vi "calc FFT_indexed.vi"(6 "#bins":i32, 7 "IQ indexes":i32[][](array[numeric]), 8 "dt":dbl=1e-06 format="%#_13g", 9 "Unit":T1, 10 "Window":T2=1 items=["Rectangle"=0, "Hanning"=1, "Hamming"=2, "Blackman-Harris"=3, "Exact Blackman"=4, "Blackman"=5, "Flat Top"=6, "4 Term B-Harris "=7, "7 Term B-Harris"=8, "Low Sidelobe"=9, "Blackman Nuttall"=11, "Triangle"=30, "Bartlett-Hanning"=31, "Bohman"=32, "Parzen"=33, "Welch"=34, "Kaiser"=60, "Dolph-Chebyshev"=61, "Gaussian"=62], 11 "data":dbl[][](array[numeric])) -> (3 "Power Spectrum / PSD":cluster{"f0":dbl, "df":dbl, "magnitude":dbl[]}[](array[cluster]) {"magnitude" format="%.2p"; "f0" format="%.2p"; "df" format="%.2p"})   [LabVIEW 2018]
uses:
  <vilib>/Analysis/4window.llb/windowTd.ctl
  controls/power_spectrum_unit.ctl
  <vilib>/measure/maspectr.llb/Power Spectrum and PSD Export Mode.ctl
  <vilib>/Analysis/0measdsp.llb/Scaled Time Domain Window (DBL).vi
  <vilib>/measure/maspectr.llb/FFT Power Spectrum and PSD for N Chan (CDB).vi
  <vilib>/measure/NI_MAPro.lvlib
  <vilib>/Analysis/NI_AALPro.lvlib
panel:
  # "each row is a pair of indexes in the data matrix.\nThe first index is I of that channelm the second is Q of that channel"
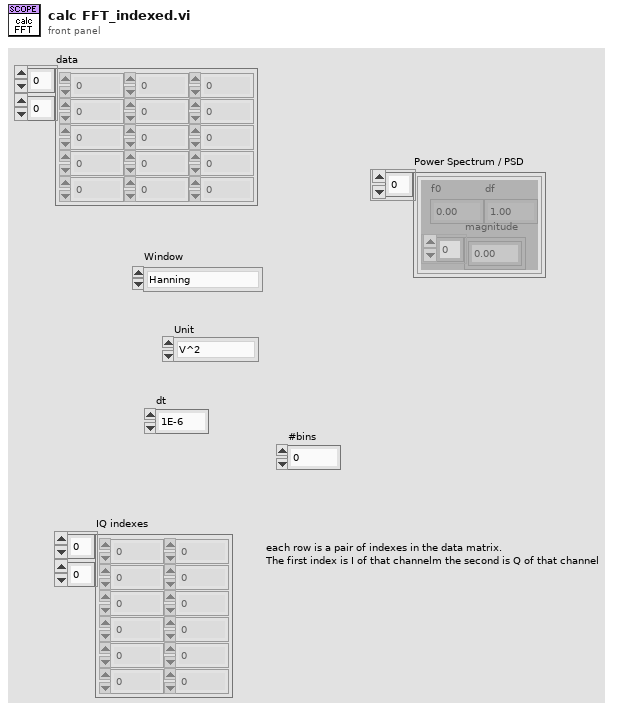
[diagram p1: front panel]
types:
  T1 = typedef "power_spectrum_unit.ctl" = enum16{"V^2", "V", "dBV"}
  T2 = typedef "NI_AALPro.lvlib/windowTd.ctl" = u32
  T3 = typedef "NI_MAPro.lvlib/Power Spectrum and PSD Export Mode.ctl" = u16
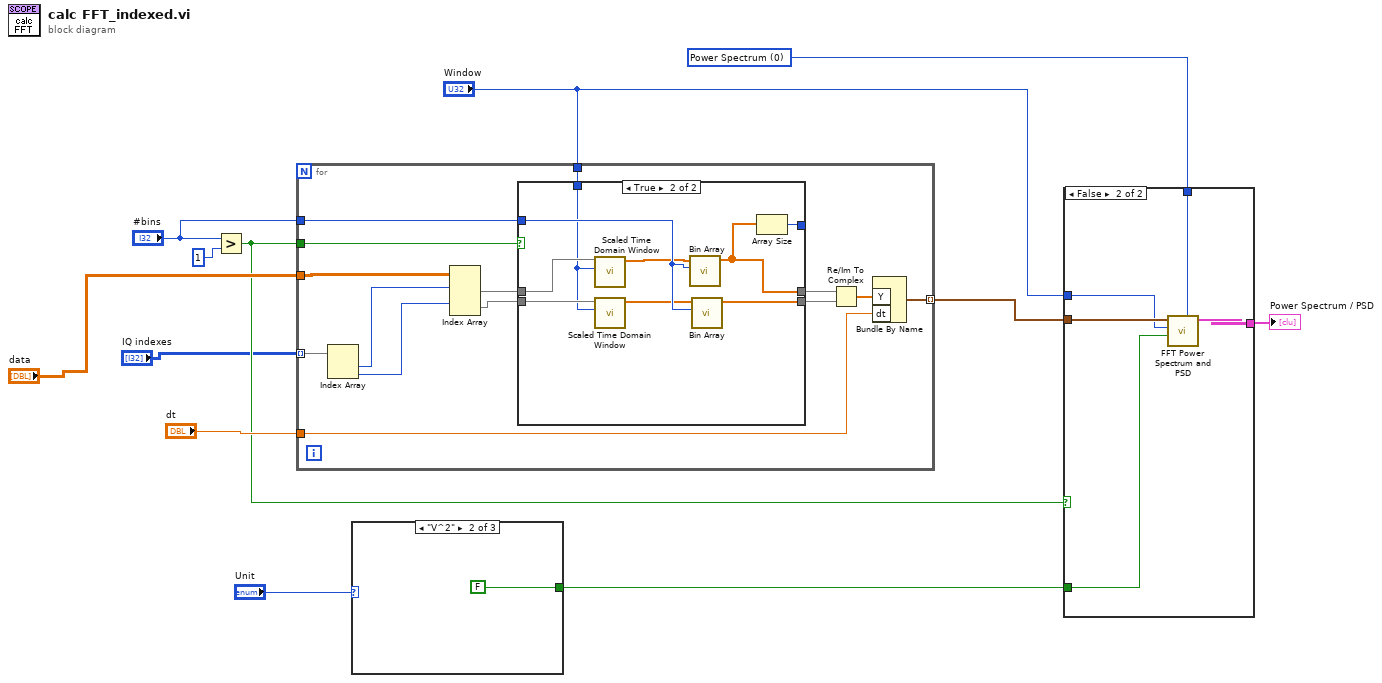
[diagram p0: block diagram]
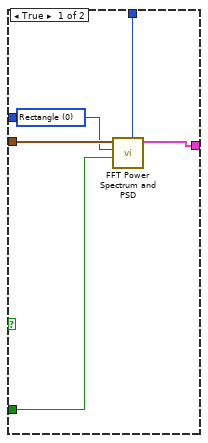
[diagram p2: hidden frame]
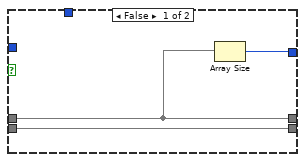
[diagram p3: hidden frame]
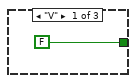
[diagram p4: hidden frame]
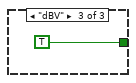
[diagram p5: hidden frame]
diagram:
  w9 = T3 0 items=["Power Spectrum", "Power Spectral Density"] ("export mode")
  n1 = Greater?(x="#bins", y=1) -> (0:w3:bool)
  n2 = for {
    tunnel: "data" -> [w26]
    tunnel: [w24] -> w6 mode=indexing
    tunnel: "dt" -> [w17]
    tunnel: w3 -> [w23]
    tunnel: "#bins" -> [w18]
    tunnel: "Window" -> [w16]
    tunnel: "IQ indexes" -> [w15] mode=indexing
    n3 = Index Array(array=w15) -> (element #1=w14:i32, element #2=w13:i32)  [unwired: 2 in]
    n4 = Index Array(array=w26, index (row) #1=w14, index (row) #2=w13) -> (element #1=w22:dbl[], element #2=w21:dbl[])  [unwired: 2 in]
    n5 = case shown="True" w23 {
      tunnel: w22 -> [w28 w34]
      tunnel: [w28 w37] -> w19
      tunnel: w21 -> [w29 w32]
      tunnel: [w29 w38] -> w20
      tunnel: w18 -> [_ w35]
      tunnel: [w27 w36] -> _
      tunnel: w16 -> [_ w31]
      frame False {
        n6 = Array Size(array=w28) -> (size(s)=w27:i32)
      }
      frame True {
        n7 = call-poly <vilib>:"Scaled Time Domain Window.vi"("window"=w31, "X"=w34) -> ("Windowed X"=w33:dbl[])  [unwired: 7 in, 2 out]
        n8 = call-poly <vilib>:"Scaled Time Domain Window.vi"("window"=w31, "X"=w32) -> ("Windowed X"=w30:dbl[])  [unwired: 7 in, 2 out]
        n9 = call "Bin Array.vi"("#bins"=w35, "Array"=w33) -> ("Binned array"=w37:dbl[])  [unwired: 9 in]
        n10 = call "Bin Array.vi"("#bins"=w35, "Array"=w30) -> ("Binned array"=w38:dbl[])  [unwired: 9 in]
        n11 = Array Size(array=w37) -> (size(s)=w36:i32)
      }
    }
    n12 = Re/Im To Complex(1:w20, 2:w19) -> (0:w25:cdb[])
    n13 = Bundle By Name("Y"=w25, "dt"=w17) -> (w24:waveform(cdb))  [unwired: 1 in]
  }
  n14 = case shown="\"V^2\"" "Unit" {
    tunnel: [FALSE ("dB On (F)") FALSE ("dB On (F)") TRUE ("dB On (F)")] -> w10
    frame "V" {
    }
    frame "V^2" {
    }
    frame "dBV" {
    }
  }
  n15 = case shown="False" w3 {
    tunnel: [w46 w51] -> w12
    tunnel: w10 -> [w45 w50]
    tunnel: w9 -> [w44 w49]
    tunnel: w6 -> [w43 w48]
    tunnel: "Window" -> [_ w47]
    frame True {
      w42 = T2 0 items=["Rectangle"=0, "Hanning"=1, "Hamming"=2, "Blackman-Harris"=3, "Exact Blackman"=4, "Blackman"=5, "Flat Top"=6, "4 Term B-Harris "=7, "7 Term B-Harris"=8, "Low Sidelobe"=9, "Blackman Nuttall"=11, "Triangle"=30, "Bartlett-Hanning"=31, "Bohman"=32, "Parzen"=33, "Welch"=34, "Kaiser"=60, "Dolph-Chebyshev"=61, "Gaussian"=62] ("window")
      n16 = call-poly <vilib>:"FFT Power Spectrum and PSD.vi"("export mode"=w44, "dB On (F)"=w45, "window"=w42, "time signals"=w43) -> ("Power Spectrum / PSD"=w46:cluster{"f0":dbl, "df":dbl, "magnitude":dbl[]}[])  [unwired: 4 in, 3 out]
    }
    frame False {
      n17 = call-poly <vilib>:"FFT Power Spectrum and PSD.vi"("export mode"=w49, "dB On (F)"=w50, "window"=w47, "time signals"=w48) -> ("Power Spectrum / PSD"=w51:cluster{"f0":dbl, "df":dbl, "magnitude":dbl[]}[])  [unwired: 4 in, 3 out]
    }
  }
  "Power Spectrum / PSD" <- w12
